vi "Hi_Port_SetTOOLt.vi"() -> ()   [LabVIEW 2018]
panel:
  out "Row":i32
  in  "Test Item":i32(listbox)
  out "Program Name:":string caption="程序名称："
  in  "TEST data":i32(listbox) caption="TEST"
  out "exit":bool
  in  "保存":bool
  in  "测试设置 2":bool
  in  "Exit":bool caption="停止"
  in  "测试设置":bool
  in  "打开编辑":bool
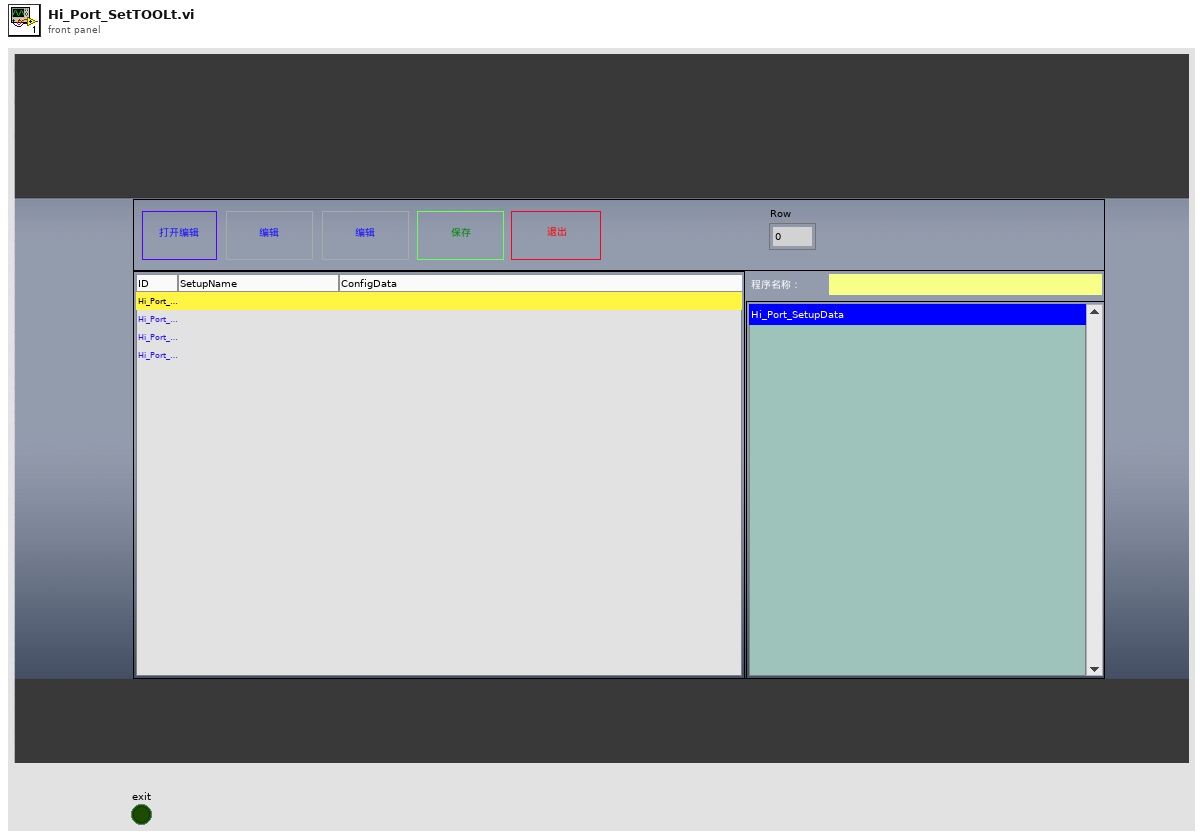
[diagram p1: front panel]
types:
  T1 = typedef "LVPoint32TypeDef.ctl" = cluster{"Horizontal":i32, "Vertical":i32}
  T2 = typedef "LVRowAndColumnTypeDef.ctl" = cluster{"Row":i32, "Column":i32}
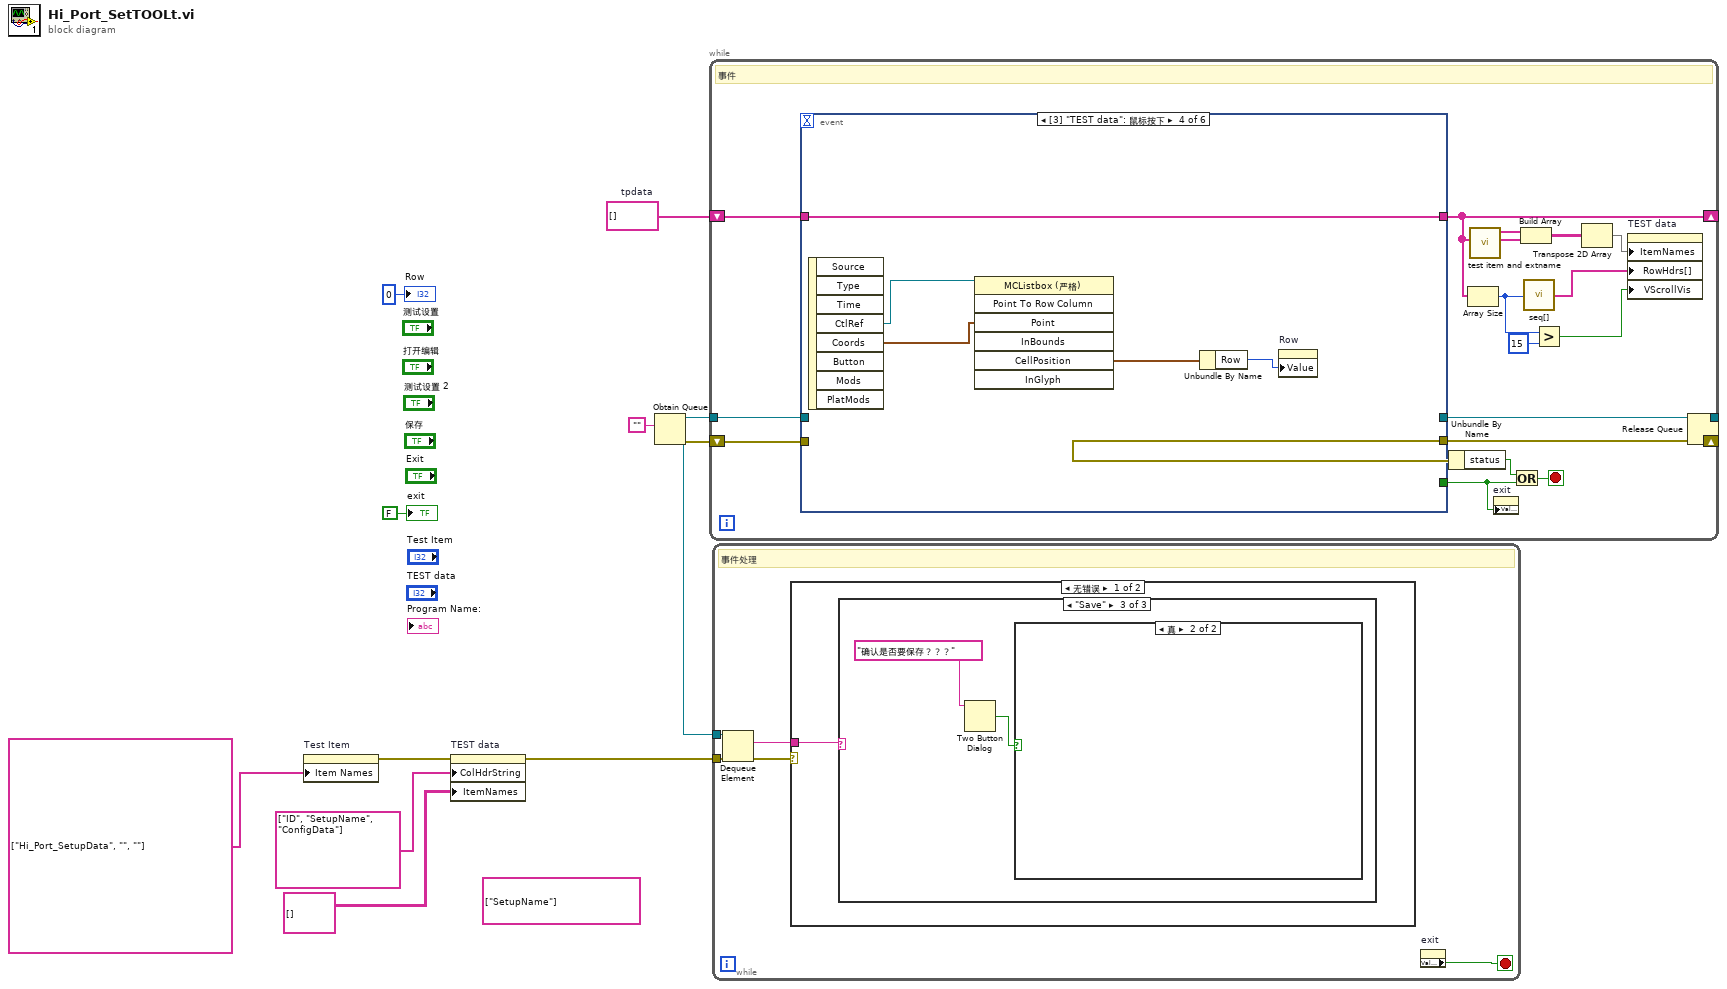
[diagram p0: block diagram]
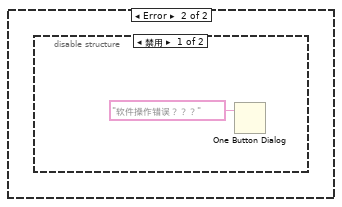
[diagram p5: hidden frame]
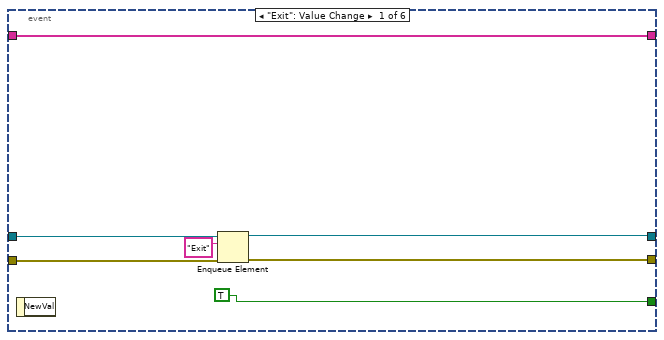
[diagram p7: hidden frame]
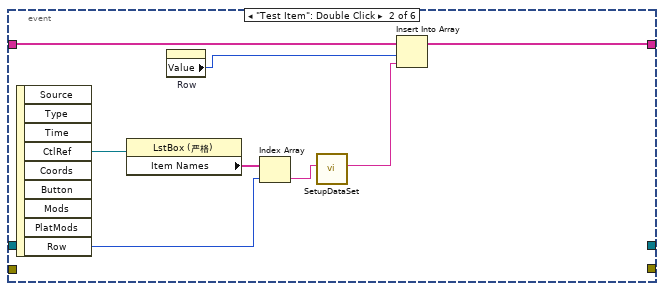
[diagram p8: hidden frame]
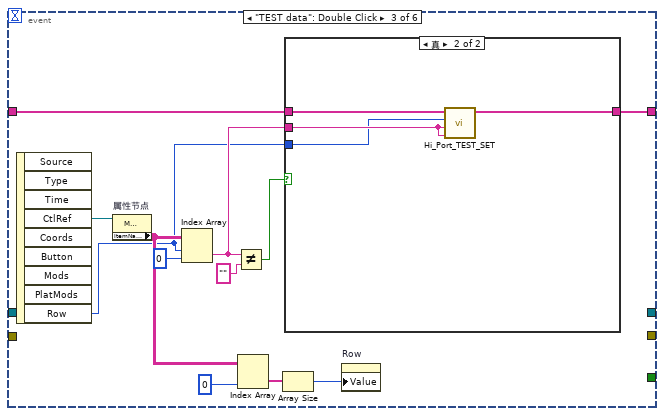
[diagram p9: hidden frame]
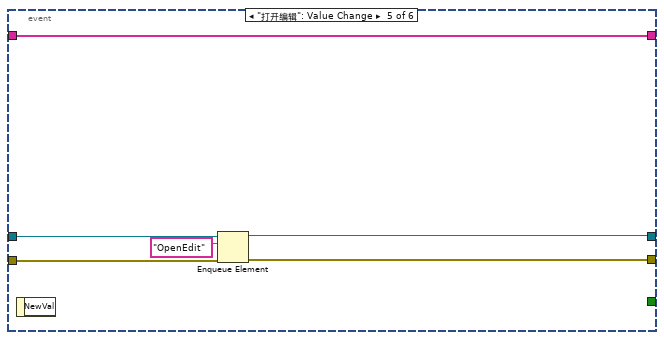
[diagram p11: hidden frame]
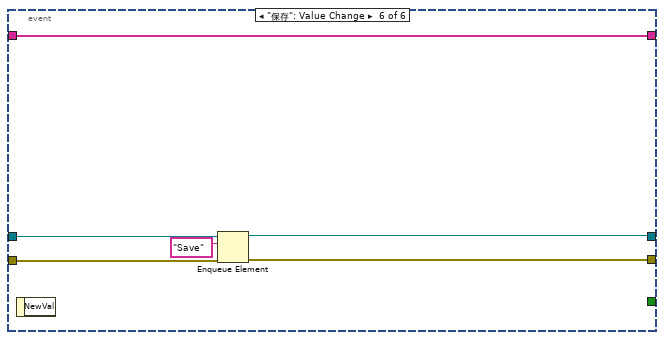
[diagram p12: hidden frame]
diagram:
  (unwired) string[] ["SetupName"]
  w2 = string[] []  # tpdata
  n1 = property on="Test Item" class="LstBox (严格)"("Item Names"=string[] ["Hi_Port_SetupData", "", ""]) -> (error out=w4:errorcluster)  [unwired: 2 in, 1 out]
  n2 = property on="TEST data" class="MCListbox (严格)"(error in=w4, "ColHdrString"=string[] ["ID", "SetupName", "ConfigData"] ("Column Header Strings[]"), "ItemNames"=string[][] [] ("项名")) -> (error out=w3:errorcluster)  [unwired: 1 in, 1 out]
  n3 = Obtain Queue(element data type="" ("数据（可为任意类型）")) -> (queue out=w13:refnum<queue>, error out=w10:errorcluster)  [unwired: 4 in, 1 out]
  n4 = while {
    shift-right: [w27] -> w11
    shift-left: w10 -> [w29]
    tunnel: w13 -> [w30]
    tunnel: [w25] -> w9
    shift-right: [w17] -> _
    shift-left: w2 -> [w23]
    stop <- w28 stop-if-true
    # "事件"
    n5 = event shown="[3] \"TEST data\": 鼠标按下" {
      selector: _ -> [_ _ _ _ _ _]
      dyn-events: _ -> [_ _ _ _ _ _]
      timeout: _ -> [_ _ _ _ _ _]
      tunnel: w30 -> [w37 _ _ _ w73 w79]
      tunnel: w29 -> [w36 _ _ _ w72 w78]
      tunnel: [w35 _ _ _ w71 w77] -> w27
      tunnel: [w33 _ _ _ w69 w75] -> w25
      tunnel: [TRUE _ _ _ _ _] -> w24
      tunnel: [w31 w41 w48 w63 w68 w74] -> w17
      tunnel: w23 -> [w31 w40 w49 w63 w68 w74]
      event "Exit": Value Change {
        n6 = event-data() -> ()  [unwired: 1 in, 1 out]
        n7 = Enqueue Element(queue=w37, element="Exit", error in (no error)=w36) -> (queue out=w33:refnum<queue>, error out=w35:errorcluster)  [unwired: 1 in, 1 out]
      }
      event "Test Item": Double Click {
        n8 = event-data() -> ("CtlRef"=w45:refnum<vi>, "Row"=w43:i32)  [unwired: 1 in, 7 out]
        n9 = property on="属性节点" class="LstBox (严格)"(reference=w45) -> ("Item Names"=w44:string[])  [unwired: 1 in, 2 out]
        n10 = property on="Row" class="DigNum (严格)"() -> ("Value"=w38:i32)  [unwired: 2 in, 2 out]
        n11 = Index Array(array=w44, index=w43) -> (element=w42:string)
        n12 = call "SetupDataSet.vi"("字符串"=w42) -> ("item data"=w39:string)  [unwired: 10 in]
        n13 = Insert Into Array(array=w40, index=w38, new element=w39) -> (w41:string[])
      }
      event "TEST data": Double Click {
        n14 = event-data() -> ("CtlRef"=w57:refnum<vi>, "Row"=w46:i32)  [unwired: 1 in, 7 out]
        n15 = property on="属性节点" class="MCListbox (严格)"(reference=w57) -> ("ItemNames"=w53:string[][])  [unwired: 1 in, 2 out]
        n16 = Index Array(array=w53, index (row)=w46, index (col)=0 ("disabled index (col)")) -> (element=w47:string)
        n17 = Not Equal?(x=w47, y="") -> (x != y?=w50:bool)
        n18 = Index Array(array=w53, index (col)=0 ("禁用的索引 (列)")) -> (element=w56:string[])  [unwired: 1 in]
        n19 = Array Size(array=w56) -> (size(s)=w52:i32)
        n20 = case shown="真" w50 {
          tunnel: w49 -> [w58 w62]
          tunnel: [w58 w61] -> w48
          tunnel: w47 -> [_ w60]
          tunnel: w46 -> [_ w59]
          frame False {
          }
          frame True {
            n21 = call "Hi_Port_TEST_SET.vi"("itemiput"=w60, "input"=w60, "SEQ"=w59, "tpdata in"=w62) -> ("tpdata out"=w61:string[])  [unwired: 3 in]
          }
        }
        n22 = property on="Row" class="DigNum (严格)"("Value"=w52) -> ()  [unwired: 2 in, 2 out]
      }
      event "TEST data": Mouse Down {
        n23 = event-data() -> ("CtlRef"=w66:refnum<vi>, "Coords"=w65:T1)  [unwired: 1 in, 6 out]
        n24 = invoke class="MCListbox (严格)" method="Point To Row Column"(reference=w66, "Point"=w65) -> ("CellPosition"=w67:T2)  [unwired: 5 in, 6 out]
        n25 = Unbundle By Name(w67) -> ("Row"=w64:i32)
        n26 = property on="Row" class="DigNum (严格)"("Value"=w64) -> ()  [unwired: 2 in, 2 out]
      }
      event "打开编辑": Value Change {
        n27 = event-data() -> ()  [unwired: 1 in, 1 out]
        n28 = Enqueue Element(queue=w73, element="OpenEdit", error in (no error)=w72) -> (queue out=w69:refnum<queue>, error out=w71:errorcluster)  [unwired: 1 in, 1 out]
      }
      event "保存": Value Change {
        n29 = event-data() -> ()  [unwired: 1 in, 1 out]
        n30 = Enqueue Element(queue=w79, element="Save", error in (no error)=w78) -> (queue out=w75:refnum<queue>, error out=w77:errorcluster)  [unwired: 1 in, 1 out]
      }
    }
    n31 = Unbundle By Name(w27) -> ("status"=w26:bool)
    n32 = Array Size(array=w17) -> (size(s)=w20:i32)
    n33 = call "test item and extname.vi"("tpdata"=w17) -> ("Nxt.Name"=w21:string[], "test item"=w22:string[])  [unwired: 9 out]
    n34 = property on="exit" class="Bool (严格)"("Value"=w24) -> ()  [unwired: 2 in, 2 out]
    n35 = Or(x=w26, y=w24) -> (x .or. y?=w28:bool)
    n36 = Build Array(w22, w21) -> (w19:string[][])
    n37 = call "seq[].vi"("数值"=w20) -> ("数组"=w16:string[])
    n38 = Greater?(x=w20, y=15) -> (0:w14:bool)
    n39 = Transpose 2D Array(2D array=w19) -> (transposed array=w15:string[][])
    n40 = property on="TEST data" class="MCListbox (严格)"("ItemNames"=w15, "RowHdrs[]"=w16, "VScrollVis"=w14) -> ()  [unwired: 2 in, 2 out]
  }
  n41 = while {
    tunnel: w13 -> [w84]
    tunnel: w3 -> [w80]
    stop <- w81 stop-if-true
    # "事件处理"
    n42 = Dequeue Element(queue=w84, error in (no error)=w80) -> (element=w82:string, error out=w83:errorcluster)  [unwired: 1 in, 2 out]
    n43 = case shown="无错误" w83 {
      tunnel: w82 -> [w85 _]
      frame No Error {
        n44 = case shown="\"Save\"" w85 {
          frame "假", Default {
          }
          frame "OpenEdit" {
          }
          frame "Save" {
            n45 = Two Button Dialog(message="确认是否要保存？？？" ("消息")) -> (T button?=w86:bool)  [unwired: 2 in]
            n46 = case shown="真" w86 {
              frame False {
              }
              frame True {
              }
            }
          }
        }
      }
      frame Error {
        n47 = disable-structure shown="禁用" {
          frame Disabled {
            n48 = One Button Dialog(message="软件操作错误？？？" ("消息")) -> ()  [unwired: 1 in, 1 out]
          }
          frame Enabled {
          }
        }
      }
    }
    n49 = property on="exit" class="Bool (严格)"() -> ("Value"=w81:bool)  [unwired: 2 in, 2 out]
  }
  n50 = Release Queue(queue=w9, error in (no error)=w11) -> ()  [unwired: 1 in, 3 out]
  "exit" <- FALSE ("exit")
  "Row" <- 0 ("Row")
